vi "SRV_Sensor PARSE_#NA.vi"(0 "Return Data":string) -> (3 "Constant Command":string, 10 "Value":u16)   [LabVIEW 2009]
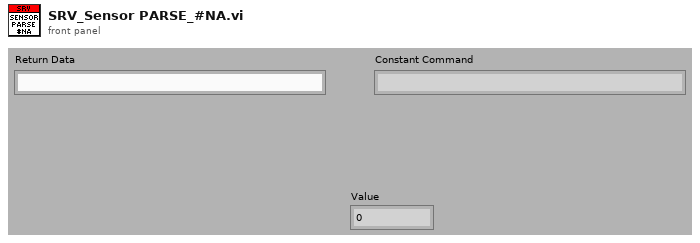
[diagram p1: front panel]
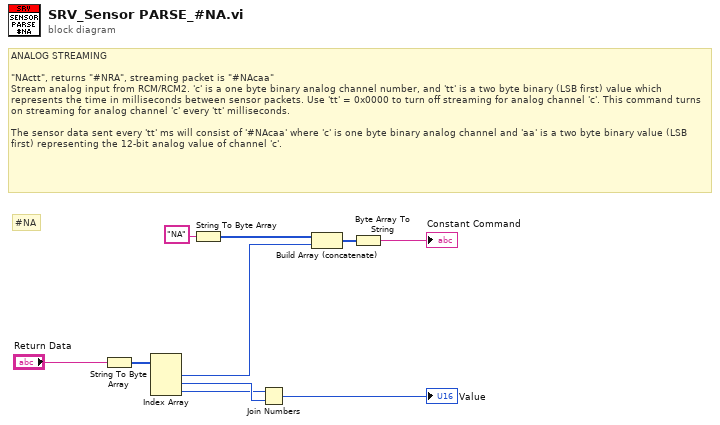
[diagram p0: block diagram]
diagram:
  # "#NA"
  # "ANALOG STREAMING\n\n\"NActt\", returns \"#NRA\", streaming packet is \"#NAcaa\"\nStream analog input from RCM/RCM2. 'c' is a one byte binary analog channel number, and 'tt' is a two byte binary (LSB first) value which represents the time in milliseconds between sensor packets. Use 'tt' = 0x0000 to turn off streaming for analog channel 'c'. This command turns on streaming for analog channel 'c' every 'tt' milliseconds.\n\nThe sensor data sent every 'tt' ms will consist of '#NAcaa' where 'c' is one byte binary analog channel and 'aa' is a two byte binary value (LSB first) representing the 12-bit analog value of channel 'c'."
  n1 = String To Byte Array(string="Return Data") -> (unsigned byte array=w5:u8[])
  n2 = Index Array(array=w5) -> (element #1=w4:u8, element #2=w3:u8, element #3=w2:u8)  [unwired: 3 in]
  n3 = String To Byte Array(string="NA" ("format string")) -> (unsigned byte array=w7:u8[])
  n4 = Join Numbers(hi=w2, lo=w3) -> ((hi.lo)=→"Value":u16)
  n5 = Build Array (concatenate)(w7, w4) -> (w10:u8[])
  n6 = Byte Array To String(unsigned byte array=w10) -> (string=→"Constant Command":string)
